vi "check if a string a whole number.vi"(11 "input string":string="0x014b4f5354414c5f") -> (3 "isAWholeNumber?":bool=TRUE)   [LabVIEW 2010]
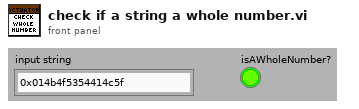
[diagram p1: front panel]
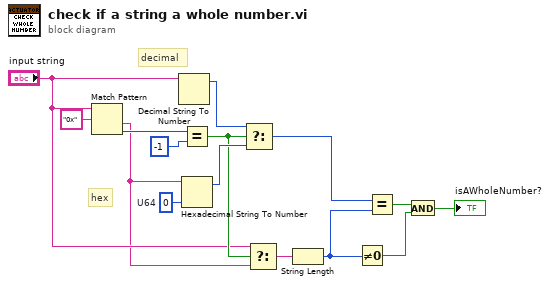
[diagram p0: block diagram]
diagram:
  w6 = u64 0  # U64
  # "hex"
  # "decimal"
  n1 = Match Pattern(string="input string", regular expression="0x") -> (after substring=w5:string, offset past match=w14:i32)  [unwired: 1 in, 2 out]
  n2 = Decimal String To Number(string="input string") -> (offset past number=w12:i32)  [unwired: 2 in, 1 out]
  n3 = Equal?(x=w14, y=-1) -> (x = y?=w10:bool)
  n4 = Hexadecimal String To Number(string=w5, default (0uL)=w6) -> (offset past number=w11:i32)  [unwired: 1 in, 1 out]
  n5 = Select(t=w12, s=w10, f=w11) -> (s? t:f=w7:i32)
  n6 = Select(t="input string", s=w10, f=w5) -> (s? t:f=w8:string)
  n7 = String Length(string=w8) -> (length=w3:i32)
  n8 = Not Equal To 0?(x=w3) -> (x != 0?=w2:bool)
  n9 = Equal?(x=w7, y=w3) -> (x = y?=w4:bool)
  n10 = And(x=w4, y=w2) -> (x .and. y?=→"isAWholeNumber?":bool)
